vi "Encode_Base_Info.vi"(8 "error in (no error)":errorcluster, 10 "Authentication Info":T1, 11 "OAuth in":refnum<class "OAuth.lvclass">) -> (0 "error out":errorcluster, 3 "OAuth out":refnum<class "OAuth.lvclass">)   [LabVIEW 2016, in "OAuth.lvclass"]
uses:
  OAuth.lvclass
  OAuth.lvclass/OAuth.ctl
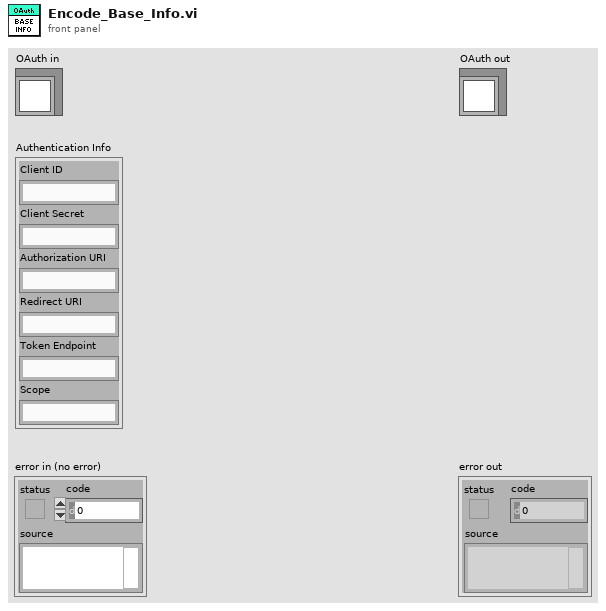
[diagram p1: front panel]
types:
  T1 = cluster{"Client ID":string, "Client Secret":string, "Authorization URI":string, "Redirect URI":string, "Token Endpoint":string, "Scope":string}
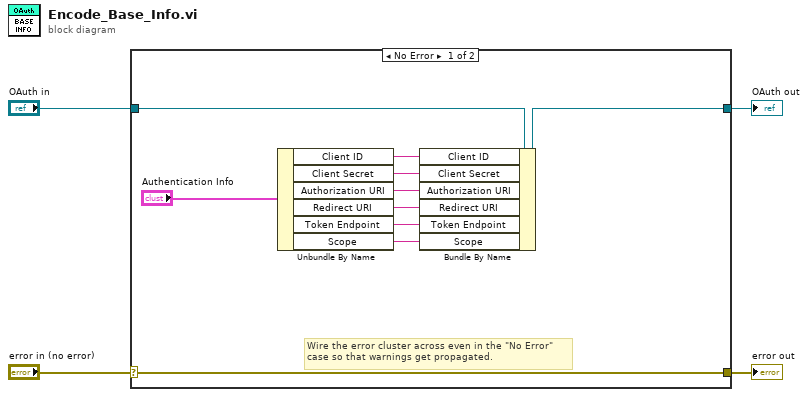
[diagram p0: block diagram]
diagram:
  n1 = case shown="No Error" "error in (no error)" {
    selector: "error in (no error)" -> [w14 w16]
    tunnel: [w14 w16] -> w3
    tunnel: [w12 w15] -> w1
    tunnel: "OAuth in" -> [w13 w15]
    frame No Error {
      # "Wire the error cluster across even in the \"No Error\"\ncase so that warnings get propagated."
      n2 = Unbundle By Name("Authentication Info") -> ("Client ID"=w5:string, "Client Secret"=w6:string, "Authorization URI"=w7:string, "Redirect URI"=w8:string, "Token Endpoint"=w9:string, "Scope"=w10:string)
      n3 = Bundle By Name(cluster=w13, "Client ID"=w5, "Client Secret"=w6, "Authorization URI"=w7, "Redirect URI"=w8, "Token Endpoint"=w9, "Scope"=w10) -> (w12:refnum<class "OAuth.lvclass">)
    }
    frame Error {
    }
  }
  "error out" <- w3
  "OAuth out" <- w1
